vi "Servo Tester.vi"() -> ()   [LabVIEW 2020]
uses:
  <vilib>/DAQmx/write.llb/DAQmx Write (Counter Frequency 1Chan 1Samp).vi
  <vilib>/DAQmx/miscellaneous.llb/DAQmx Fill In Error Info.vi
panel:
  in  "stop":bool
  in  "frequency":dbl=300.0 format="%#_13g"
  in  "duty cycle":dbl=5.0 format="%_6g"
  in  "task/channels in":refnum<k21>
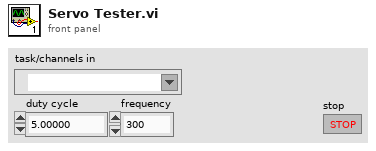
[diagram p1: front panel]
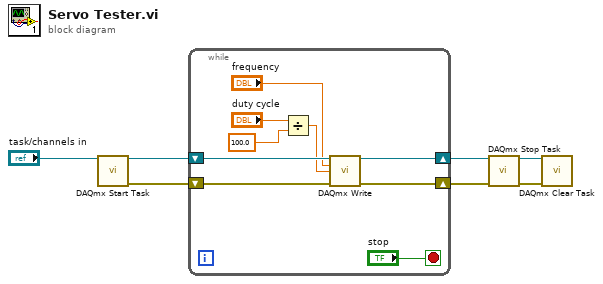
[diagram p0: block diagram]
diagram:
  n1 = call <vilib>:"DAQmx Start Task.vi"("task/channels in"="task/channels in") -> ("task out"=w4:refnum<k21>, "error out"=w3:errorcluster)  [unwired: 13 in]
  n2 = while {
    shift-right: [w12] -> w1
    shift-left: w4 -> [w16]
    shift-right: [w13] -> w2
    shift-left: w3 -> [w15]
    stop <- "stop" stop-if-true
    n3 = Divide(x="duty cycle", y=100.0) -> (x/y=w9:dbl)
    n4 = call-poly <vilib>:"DAQmx Write.vi"("task/channels in"=w16, "frequency"="frequency", "duty cycle"=w9, "error in"=w15) -> ("task out"=w12:refnum<k21>, "error out"=w13:errorcluster)  [unwired: 9 in, 1 out]
  }
  n5 = call <vilib>:"DAQmx Stop Task.vi"("task/channels in"=w1, "error in"=w2) -> ("task out"=w5:refnum<k21>, "error out"=w6:errorcluster)  [unwired: 12 in]
  n6 = call <vilib>:"DAQmx Clear Task.vi"("task in"=w5, "error in"=w6) -> ()  [unwired: 13 in, 1 out]
